vi "Check for Fresh Message.vi"(8 "error in":errorcluster, 11 "Handle PAS Voffset Request in":refnum<class "Handle PAS Voffset Request.lvclass">) -> (0 "error out":errorcluster, 1 "Enqueuer":refnum<class "Message Enqueuer.lvclass">, 2 "Enqueuer not Valid":bool, 3 "Handle PAS Voffset Request out":refnum<class "Handle PAS Voffset Request.lvclass">)   [LabVIEW 2014, in "Handle PAS Voffset Request.lvclass"]
doc: "This method is a dynamic method that \n1) checks for a good connection to the shared variable. If it is not present, then it attempts to connect If a connection is not available, then this VI will do nothing.\n2) Check the state of the enqueuer. If the state is no good, return with this indication and do nothing.\n2) If the connection is good, check to see if the current shared variable state has changed.\n3) If the state has changed, pump the message into the appropriate enqueuer."
uses:
  Handle PAS Voffset Request.lvclass
  <vilib>/ActorFramework/Message Enqueuer/Message Enqueuer.lvclass
  Instr Actor/Messages/Set Voffset MSG/Set Voffset MSG.lvclass
  Instr Actor/Messages/Set Voffset MSG/Set Voffset MSG.lvclass/Set Voffset MSG.ctl
  <vilib>/ActorFramework/Message Enqueuer/Message Enqueuer.lvclass/Message Enqueuer.ctl
  Instr Actor/Messages/Set Voffset MSG/Write Voffset.vi
  <vilib>/ActorFramework/Message Priority Queue/Priority Enqueue.vi
  Network Command Processor.lvclass
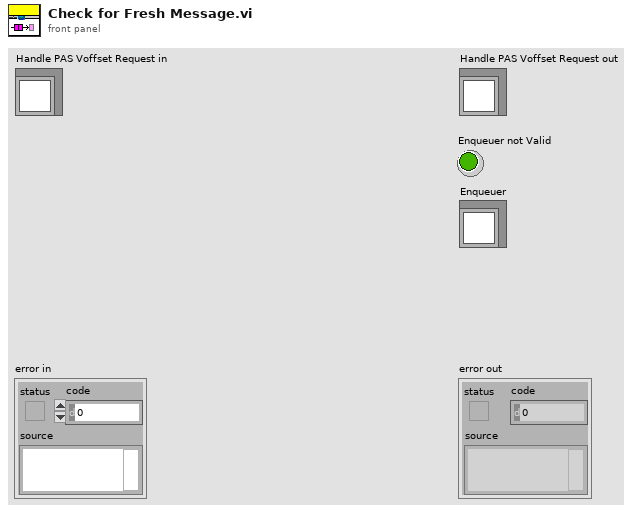
[diagram p1: front panel]
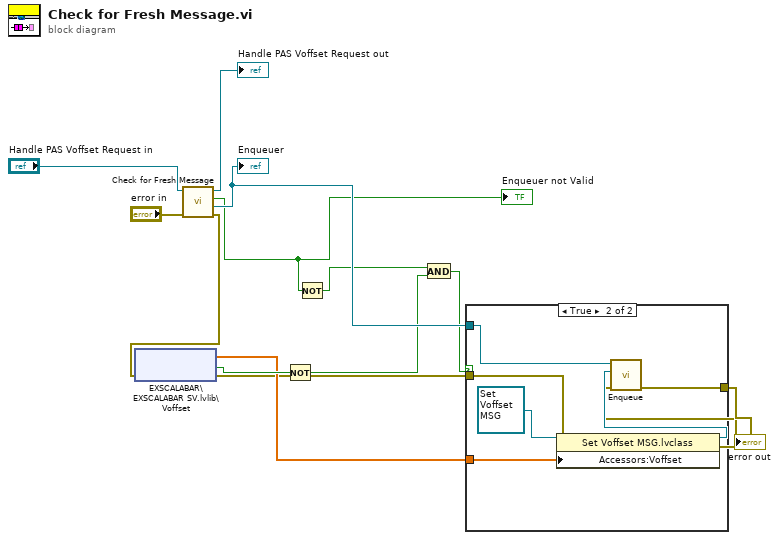
[diagram p0: block diagram]
diagram:
  n1 = call-parent "Check for Fresh Message.vi"("error in"="error in", "Network Command Processor in"="Handle PAS Voffset Request in") -> ("error out"=w3:errorcluster, "Enqueuer"=w10:refnum<class "Message Enqueuer.lvclass">, "Enqueuer not Valid"=w8:bool, "Network Command Processor out"=→"Handle PAS Voffset Request out":refnum<class "Handle PAS Voffset Request.lvclass">)  [unwired: 6 in]
  "Enqueuer not Valid" <- w8
  "Enqueuer" <- w10
  n2 = shared-variable "EXSCALABAR\\EXSCALABAR SV.lvlib\\Voffset"(error in=w3) -> (w4:sgl[], error out=w2:errorcluster, w9:bool)  [unwired: 1 in]
  n3 = Not(x=w9) -> (.not. x?=w6:bool)
  n4 = Not(x=w8) -> (.not. x?=w7:bool)
  n5 = And(x=w7, y=w6) -> (x .and. y?=w5:bool)
  n6 = case shown="True" w5 {
    tunnel: w10 -> [_ w19]
    tunnel: w4 -> [_ w21]
    tunnel: w2 -> [w14 w18]
    tunnel: [w14 w16] -> w1
    frame False {
    }
    frame True {
      n7 = property class="Set Voffset MSG.lvclass"(reference=refnum<class "Set Voffset MSG.lvclass"> refnum ("Instrument Lib:Set Voffset MSG.lvclass"), error in=w18, "Accessors:Voffset"=w21) -> (reference out=w20:refnum<class "Set Voffset MSG.lvclass">, error out=w17:errorcluster)
      n8 = call <vilib>:"Enqueue.vi"("error in (no error)"=w17, "Message"=w20, "Message Enqueuer in"=w19) -> ("error out"=w16:errorcluster)  [unwired: 7 in, 1 out]
    }
  }
  "error out" <- w1
